vi "Parse SSH_FXP_STATUS.vi"(8 "error in":errorcluster, 11 "payload":u8[](array[numeric])) -> (0 "error out":errorcluster, 1 "language tag":string, 2 "error message":string, 3 "error/status code":T1)   [LabVIEW 2020, in "NI_SFTP.lvlib"]
uses:
  <vilib>/net/SFTP/NI_SFTP.lvlib
  <vilib>/net/SFTP/Low Level Connection/Status Code.ctl
  f023bfa8-f8fb-3feb-c0fc-b0554016e43f.vi
  fe9cab8e-2cf0-3fe7-1c9b-f8983c6ade3f.vi
  248d59e0-ee9f-3fd5-30f8-f80d1baee43f.vi
  <vilib>/Bit Manipulation/Network-Order Bytes To Words Poly.vi
  <vilib>/Bit Manipulation/wrappers/Network-Order Bytes To Words/Network-Order Bytes To Words U32.vi
  <vilib>/net/SFTP/Low Level Connection/Low Level Connection.lvclass
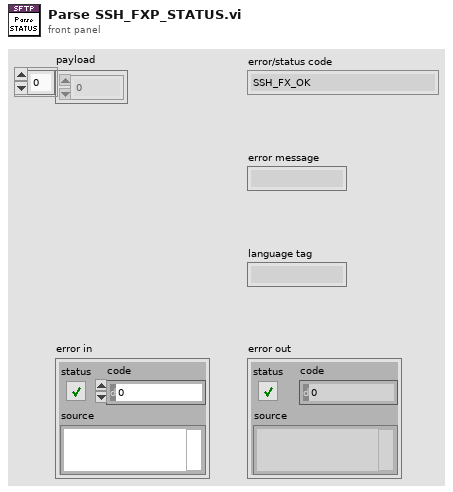
[diagram p1: front panel]
types:
  T1 = typedef "NI_SFTP.lvlib/Low Level Connection.lvclass/Status Code.ctl" = enum32{"SSH_FX_OK", "SSH_FX_EOF", "SSH_FX_NO_SUCH_FILE", "SSH_FX_PERMISSION_DENIED", "SSH_FX_FAILURE", "SSH_FX_BAD_MESSAGE", "SSH_FX_OP_UNSUPPORTED"}
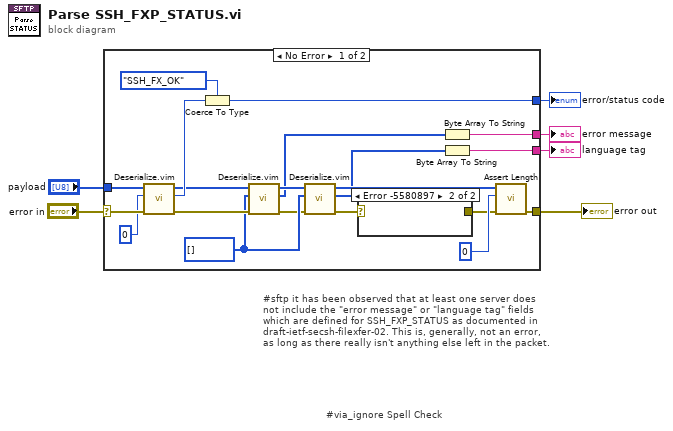
[diagram p0: block diagram]
diagram:
  # "#via_ignore Spell Check"
  # "#sftp it has been observed that at least one server does not include the \"error message\" or \"language tag\" fields which are defined for SSH_FXP_STATUS as documented in draft-ietf-secsh-filexfer-02. This is, generally, not an error, as long as there really isn't anything else left in the packet."
  n1 = case shown="No Error" "error in" {
    selector: "error in" -> [w25 w28]
    tunnel: [w22 w28] -> w5
    tunnel: "payload" -> [w26 _]
    tunnel: [w10 _] -> w1
    tunnel: [w12 _] -> w2
    tunnel: [w19 _] -> w3
    frame No Error {
      w14 = u8[] [] ("Array")
      n2 = call "Deserialize.vim"("error in"=w25, "type"=u32 0, "bytes"=w26) -> ("error out"=w24:errorcluster, "value"=w20:u32, "remaining bytes"=w16:u8[])  [unwired: 6 in]
      n3 = Coerce To Type(0:w20, 1:Status_Code."SSH_FX_OK" ("Status Code")) -> (2:w19:T1)
      n4 = call "Deserialize.vim"("error in"=w24, "type"=w14, "bytes"=w16) -> ("error out"=w7:errorcluster, "value"=w13:u8[], "remaining bytes"=w15:u8[])  [unwired: 6 in]
      n5 = call "Deserialize.vim"("error in"=w7, "type"=w14, "bytes"=w15) -> ("error out"=w9:errorcluster, "value"=w11:u8[], "remaining bytes"=w17:u8[])  [unwired: 6 in]
      n6 = case shown="Error -5580897" w9 {
        selector: w9 -> [w27 _]
        tunnel: [w27 _] -> w8
        frame #0 {
        }
        frame #1 {
        }
      }
      n7 = Byte Array To String(unsigned byte array=w13) -> (string=w12:string)
      n8 = Byte Array To String(unsigned byte array=w11) -> (string=w10:string)
      n9 = call <vilib>:"Assert Length.vi"("error in"=w8, "asserted length"=u32 0, "string in"=w17) -> ("error out"=w22:errorcluster)  [unwired: 7 in, 1 out]
    }
    frame Error {
    }
  }
  "error out" <- w5
  "error/status code" <- w3
  "error message" <- w2
  "language tag" <- w1
